vi "sensor cmd error log get.vi"(9 "error_id":u16, 10 "offset":u16, 11 "device_handle":u32) -> (1 "error_id out":u16, 2 "function return":i32, 3 "device_handle out":u32)   [LabVIEW 2019, in "apdm.lvlib"]
doc: "APDM_EXPORT int apdm_sensor_cmd_error_log_get(apdm_device_handle_t device_handle, const uint16_t offset, uint16_t *error_id);"
uses:
  apdm.lvlib
  Lee Lab/CP FES Walking 2018/Code/Working/LabVIEW/apdm.dll
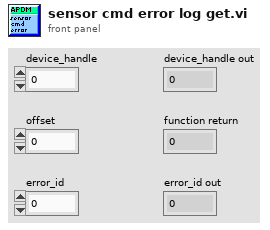
[diagram p1: front panel]
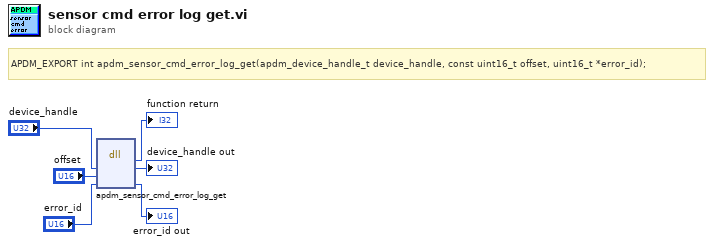
[diagram p0: block diagram]
diagram:
  # "APDM_EXPORT int apdm_sensor_cmd_error_log_get(apdm_device_handle_t device_handle, const uint16_t offset, uint16_t *error_id);"
  n1 = dll-call lib="C:/Users/jfalesi/Dropbox/Lee Lab/CP FES Walking 2018/Code/Working/LabVIEW/apdm.*" fn="apdm_sensor_cmd_error_log_get"("device_handle"="device_handle", "offset"="offset", "error_id"="error_id") -> (→"function return":i32, "device_handle"=→"device_handle out":u32, "error_id"=→"error_id out":u16)  [unwired: 4 in, 2 out]
